vi "http free response.vi"(8 "error in (no error)":errorcluster, 11 "handle":u64) -> (0 "error out":errorcluster, 2 "function return":i32, 3 "handle out":u64)   [LabVIEW 2020, in "reqwest-labview.lvlib"]
doc: "int http_free_response(void *handle);"
uses:
  reqwest-labview.lvlib
  lib_reqwest_labview_64.dll
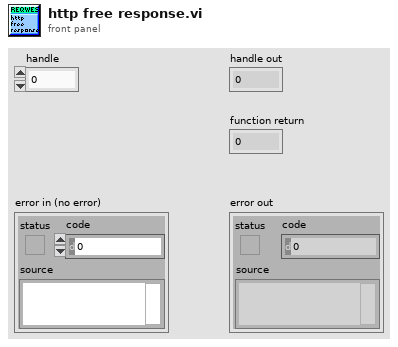
[diagram p1: front panel]
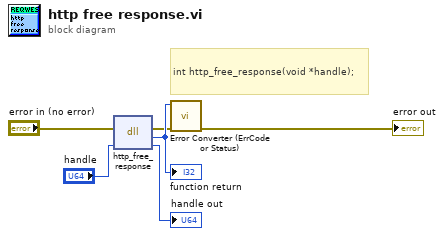
[diagram p0: block diagram]
diagram:
  # "int http_free_response(void *handle);"
  n1 = dll-call lib="C:/code/reqwest-labview/lv-src/shared-library/lib_reqwest_labview_*.*" fn="http_free_response"(error in="error in (no error)", "handle"="handle") -> (error out=w2:errorcluster, "return type"=w6:i32, "handle"=→"handle out":u64)  [unwired: 2 in, 1 out]
  "function return" <- w6
  n2 = call "Error Converter (ErrCode or Status).vi"("error in (no error)"=w2, "error code"=w6) -> ("error out"=→"error out":errorcluster)  [unwired: 9 in]
